vi "set_image_processor.vi"(8 "error in (no error)":errorcluster, 10 "image processor":refnum<class "GenericImageProcessor.lvclass">, 11 "GenericImageProcessorChangedCommand.lvclass in":refnum<class "GenericImageProcessorChangedCommand.lvclass">) -> (0 "error out":errorcluster, 3 "GenericImageProcessorChangedCommand.lvclass out":refnum<class "GenericImageProcessorChangedCommand.lvclass">)   [LabVIEW 2010, in "GenericImageProcessorChangedCommand.lvclass"]
uses:
  GenericImageProcessorChangedCommand.lvclass
  ImageProcessor/GenericImageProcessor/GenericImageProcessor/GenericImageProcessor.lvclass
  GenericImageProcessorChangedCommand.lvclass/GenericImageProcessorChangedCommand.ctl
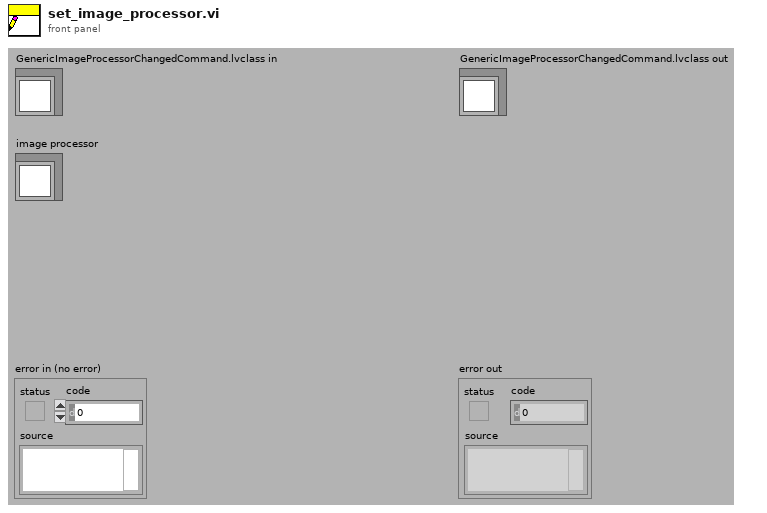
[diagram p1: front panel]
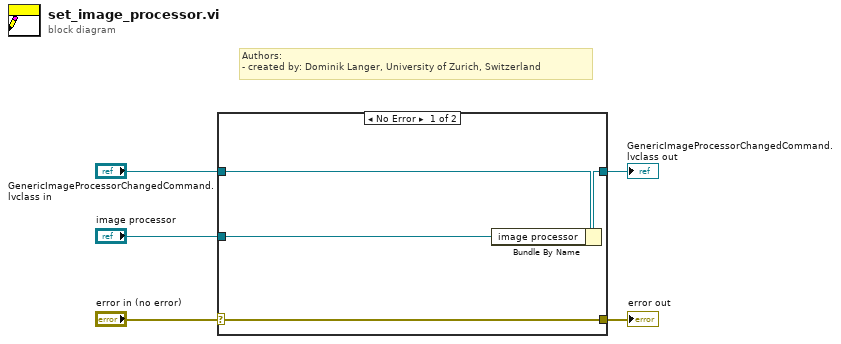
[diagram p0: block diagram]
diagram:
  # "Authors: \n- created by: Dominik Langer, University of Zurich, Switzerland"
  n1 = case shown="No Error" "error in (no error)" {
    selector: "error in (no error)" -> [w9 w10]
    tunnel: [w9 w10] -> w4
    tunnel: [w7 w11] -> w2
    tunnel: "GenericImageProcessorChangedCommand.lvclass in" -> [w8 w11]
    tunnel: "image processor" -> [w6 _]
    frame No Error {
      n2 = Bundle By Name(cluster=w8, "image processor"=w6) -> (w7:refnum<class "GenericImageProcessorChangedCommand.lvclass">)
    }
    frame Error {
    }
  }
  "error out" <- w4
  "GenericImageProcessorChangedCommand.lvclass out" <- w2
